vi "11.1.1.-SubVI Entrenamiento de Neurona Perceptrón.vi"(9 "X2":dbl[](array[numeric]), 10 "X1":dbl[](array[numeric]), 11 "T = Umbral de Activación":dbl[](array[numeric])) -> (1 "W1":dbl, 2 "W2":dbl, 3 "B = Bias":dbl)   [LabVIEW 2020]
panel:
  # "Visión Artificial - Entrenamiento Neuronal - Neurona Perceptron\nDiego Cervantes Rodríguez\ndicer0.com"
  # "Función de Agregación de la Neurona Perceptrón = Suma Ponderada = Sp = sum(wi*xi)+b = sum(w1*x1+w2*x2)+b"
  # "Función de Activación de la Neurona Perceptrón = f(x) = 1 cuando Sp > 0;  f(x) = 0 cuando Sp < 0"
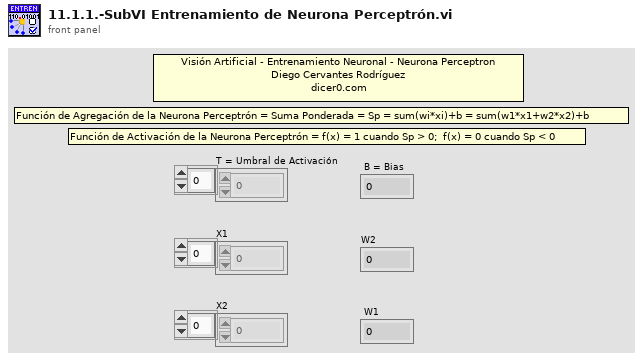
[diagram p1: front panel]
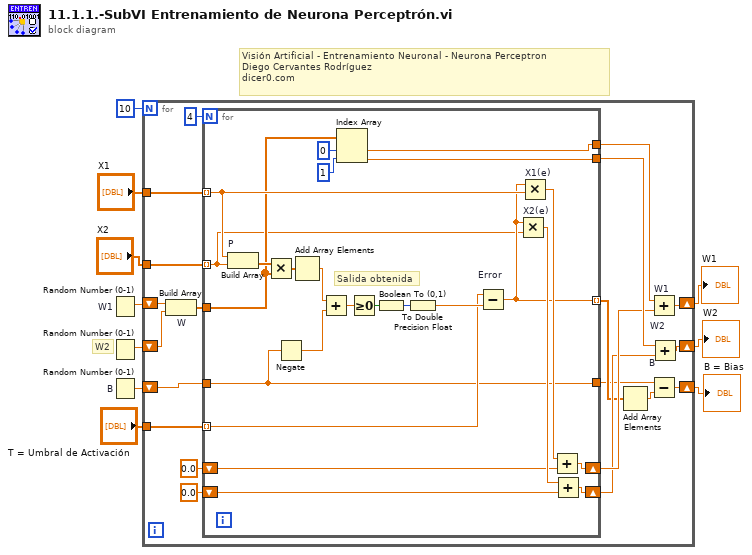
[diagram p0: block diagram]
diagram:
  # "Visión Artificial - Entrenamiento Neuronal - Neurona Perceptron\nDiego Cervantes Rodríguez\ndicer0.com"
  # "W2"
  n1 = Random Number (0-1) "W1"() -> (number: 0 to 1=w3:dbl)
  n2 = Random Number (0-1)() -> (number: 0 to 1=w1:dbl)
  n3 = Random Number (0-1) "B"() -> (number: 0 to 1=w2:dbl)
  n4 = for {
    N: 10 -> [_]
    tunnel: "X1" -> [w30]
    tunnel: "X2" -> [w29]
    tunnel: "T = Umbral de Activación" -> [w27]
    shift-right: [w26] -> w8
    shift-left: w2 -> [w28]
    shift-right: [w19] -> w9
    shift-left: w3 -> [w25]
    shift-right: [w18] -> w10
    shift-left: w1 -> [w24]
    n5 = Build Array "W"(w25, w24) -> (w23:dbl[])
    n6 = for {
      N: 4 -> [_]
      tunnel: w23 -> [w46]
      tunnel: w30 -> [w47] mode=indexing
      tunnel: w29 -> [w32] mode=indexing
      tunnel: w28 -> [w33]
      tunnel: w27 -> [w34] mode=indexing
      tunnel: [w33] -> w14
      tunnel: [w43] -> w11
      tunnel: [w31] -> w22
      shift-right: [w40] -> w17
      shift-left: 0.0 -> [w38]
      shift-right: [w39] -> w16
      shift-left: 0.0 -> [w37]
      tunnel: [w36] -> w15 mode=indexing
      # "Salida obtenida"
      n7 = Build Array "P"(w47, w32) -> (w50:dbl[])
      n8 = Multiply(x=w50, y=w46) -> (x*y=w49:dbl[])
      n9 = Negate(x=w33) -> (-x=w54:dbl)
      n10 = Add Array Elements(numeric array=w49) -> (sum=w48:dbl)
      n11 = Add(x=w48, y=w54) -> (x+y=w53:dbl)
      n12 = Index Array "Index Array"(array=w46, index #1=0 ("index"), index #2=1 ("index")) -> (element #1=w43:dbl, element #2=w31:dbl)
      n13 = Greater Or Equal To 0?(x=w53) -> (x >= 0?=w52:bool)
      n14 = Boolean To (0,1)(Boolean=w52) -> (0, 1=w51:i16)
      n15 = To Double Precision Float(number=w51) -> (double precision float=w35:dbl)
      n16 = Subtract "Error"(x=w34, y=w35) -> (x-y=w36:dbl)
      n17 = Multiply "X2(e)"(x=w36, y=w32) -> (x*y=w41:dbl)
      n18 = Multiply "X1(e)"(x=w36, y=w47) -> (x*y=w42:dbl)
      n19 = Add(x=w42, y=w38) -> (x+y=w40:dbl)
      n20 = Add(x=w41, y=w37) -> (x+y=w39:dbl)
    }
    n21 = Add Array Elements(numeric array=w15) -> (sum=w12:dbl)
    n22 = Add "W1"(x=w11, y=w17) -> (x+y=w19:dbl)
    n23 = Subtract "B"(x=w14, y=w12) -> (x-y=w26:dbl)
    n24 = Add "W2"(x=w22, y=w16) -> (x+y=w18:dbl)
  }
  "W2" <- w10
  "W1" <- w9
  "B = Bias" <- w8
